vi "init_parameters.vi"() -> (3 "Resource name out":string)   [LabVIEW 2019, in "dummyCam.lvclass"]
uses:
  dummyCam.lvclass
panel:
  in  "continue":bool
  in  "Resource name":string="dummy cam"
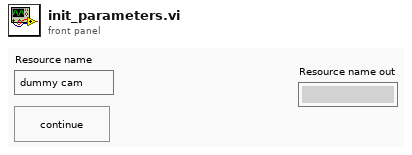
[diagram p1: front panel]
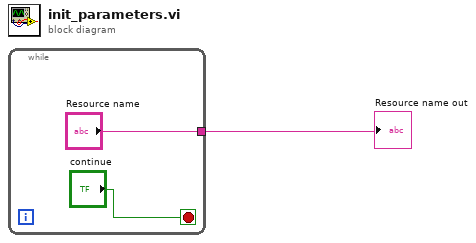
[diagram p0: block diagram]
diagram:
  n1 = while {
    tunnel: ["Resource name"] -> w1
    stop <- "continue" stop-if-true
  }
  "Resource name out" <- w1
